vi "getVideoModesAndAtrributes.vi"(8 "error in (no error)":errorcluster, 11 "HGF_IMAQDevice in":refnum<class "HGF_IMAQDevice.lvclass">) -> (0 "error out":errorcluster, 1 "Attribute Information":T2(array[cluster]), 2 "Video Modes":T3(array[cluster]), 3 "HGF_IMAQDevice out":refnum<class "HGF_IMAQDevice.lvclass">, 4 "Attribute Names":string[](array[string]))   [LabVIEW 2014, in "HGF_IMAQ.lvlib" / "HGF_IMAQDevice.lvclass"]
doc: "Get available Video Modes and Attribute Informations."
uses:
  HGF_IMAQDevice.lvclass
  <vilib>/vision/driver/IMAQdx.llb/IMAQdx Attribute Type.ctl
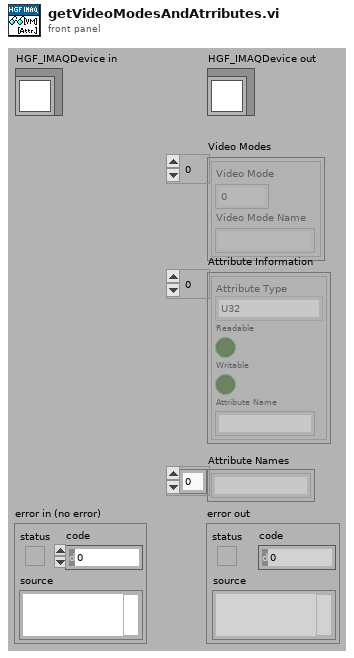
[diagram p1: front panel]
types:
  T1 = typedef "NI_Vision_Acquisition_Software.lvlib/IMAQdx Attribute Type.ctl" = enum32{"U32", "I64", "DBL", "String", "Enum", "Bool", "Command"}
  T2 = cluster{"Attribute Type":T1, "Readable":bool, "Writable":bool, "Attribute Name":string}[]
  T3 = cluster{"Video Mode":u32, "Video Mode Name":string}[]
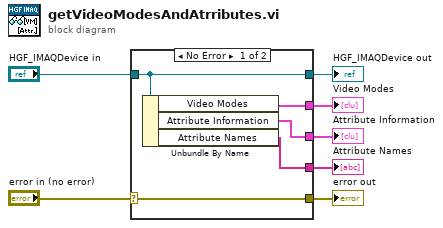
[diagram p0: block diagram]
diagram:
  n1 = case shown="No Error" "error in (no error)" {
    selector: "error in (no error)" -> [w12 w13]
    tunnel: [w12 w13] -> w6
    tunnel: [w11 w14] -> w4
    tunnel: "HGF_IMAQDevice in" -> [w11 w14]
    tunnel: [w10 _] -> w3
    tunnel: [w9 _] -> w2
    tunnel: [w8 _] -> w1
    frame No Error {
      n2 = Unbundle By Name(w11) -> ("Video Modes"=w10:T3, "Attribute Information"=w9:T2, "Attribute Names"=w8:string[])
    }
    frame Error {
    }
  }
  "error out" <- w6
  "HGF_IMAQDevice out" <- w4
  "Video Modes" <- w3
  "Attribute Information" <- w2
  "Attribute Names" <- w1
